vi "Reorder elements.vi"(8 "error in (no error)":errorcluster, 10 "Data Variant":variant, 11 "Reference Variant":variant) -> (0 "error out":errorcluster, 3 "Output VData":variant)   [LabVIEW 2015]
uses:
  <vilib>/Utility/Data Type/NI_Data Type.lvlib
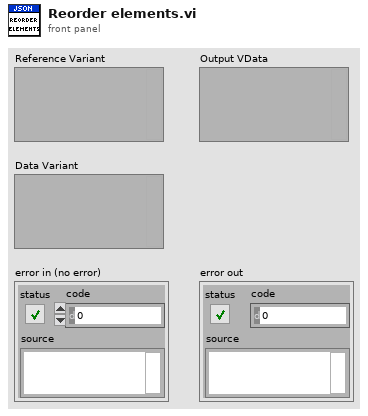
[diagram p1: front panel]
types:
  T1 = typedef "NI_Data Type.lvlib/Data Type.ctl" = enum8{"Invalid Type", "Void", "I8", "I16", "I32", "I64", "U8", "U16", "U32", "U64", "Single Float", "Double Float", "Extended Float", "Single Complex", "Double Complex", "Extended Complex", "Enum U8", "Enum U16", "Enum U32", "Enum U64", "Single Float With Unit", "Double Float With Unit", "Extended Float With Unit", "Single Complex with Unit", "Double Complex with Unit", "Extended Complex with Unit", "Boolean", "String", "Path", "Picture", "Tag", "Array", "Cluster", "Variant", "LV Variant", "Waveform", "Timestamp", "Digital Waveform", "Digital Data", "ExpressData", "Refnum", "External Data", "VI", "Poly VI", "LabVIEW Class Instance", "Fixed Point"}
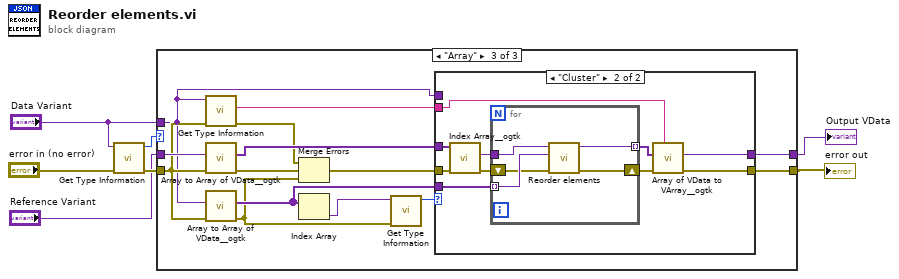
[diagram p0: block diagram]
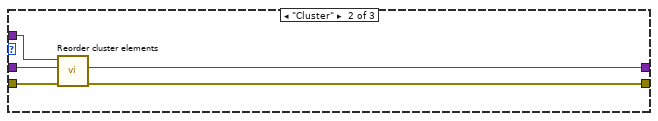
[diagram p3: hidden frame]
diagram:
  n1 = call <vilib>:"Get Type Information.vi"("error in (no error)"="error in (no error)", "Variant"="Data Variant") -> ("error out"=w7:errorcluster, "Type"=w6:T1)  [unwired: 5 in, 3 out]
  n2 = case shown="\"Array\"" w6 {
    tunnel: "Data Variant" -> [w9 w14 w16]
    tunnel: "Reference Variant" -> [_ w13 w28]
    tunnel: w7 -> [w8 w12 w23]
    tunnel: [w8 w11 w20] -> w2
    tunnel: [w9 w10 w21] -> w1
    frame Default {
    }
    frame "Cluster" {
      n3 = call "Reorder cluster elements.vi"("error in (no error)"=w12, "Reference Variant"=w13, "Data Variant"=w14) -> ("error out"=w11:errorcluster, "Ordered VCluster"=w10:variant)  [unwired: 4 in, 3 out]
    }
    frame "Array" {
      n4 = call <vilib>:"Get Type Information.vi"("error in (no error)"=w23, "Variant"=w16) -> ("error out"=w22:errorcluster, "Name"=w24:string)  [unwired: 5 in, 3 out]
      n5 = call <userlib>:"Array to Array of VData__ogtk.vi"("error in (no error)"=w23, "MultiD Array"=w28) -> ("error out"=w26:errorcluster, "1D Array of Variants"=w27:variant[])  [unwired: 8 in]
      n6 = call <userlib>:"Array to Array of VData__ogtk.vi"("error in (no error)"=w23, "MultiD Array"=w16) -> ("error out"=w17:errorcluster, "1D Array of Variants"=w19:variant[])  [unwired: 8 in]
      n7 = Merge Errors(w22, w26, w17) -> (w25:errorcluster)
      n8 = Index Array(array=w19) -> (element=w18:variant)  [unwired: 1 in]
      n9 = call <vilib>:"Get Type Information.vi"("error in (no error)"=w17, "Variant"=w18) -> ("Type"=w15:T1)  [unwired: 5 in, 4 out]
      n10 = case shown="\"Cluster\"" w15 {
        tunnel: w27 -> [_ w40]
        tunnel: w25 -> [w29 w38]
        tunnel: w24 -> [_ w36]
        tunnel: [w30 w35] -> w21
        tunnel: [w29 w34] -> w20
        tunnel: w19 -> [_ w32]
        tunnel: w16 -> [w30 _]
        frame "Invalid Type", Default {
        }
        frame "Cluster" {
          n11 = call <userlib>:"Index Array__ogtk.vi"("error in (no error)"=w38, "MultiD Array"=w40) -> ("error out"=w31:errorcluster, "Array Element"=w39:variant)  [unwired: 8 in]
          n12 = for {
            tunnel: w39 -> [w43]
            tunnel: w32 -> [w44] mode=indexing
            shift-right: [w41] -> w37
            shift-left: w31 -> [w42]
            tunnel: [w45] -> w33 mode=indexing
            n13 = call "Reorder elements.vi"("error in (no error)"=w42, "Data Variant"=w44, "Reference Variant"=w43) -> ("error out"=w41:errorcluster, "Output VData"=w45:variant)  [unwired: 7 in]
          }
          n14 = call <userlib>:"Array of VData to VArray__ogtk.vi"("Array Name"=w36, "error in (no error)"=w37, "1D Array of VData"=w33) -> ("error out"=w34:errorcluster, "VArray"=w35:variant)  [unwired: 7 in]
        }
      }
    }
  }
  "error out" <- w2
  "Output VData" <- w1
